vi "Read Servicio Seleccionado.vi"(8 "error in (no error)":errorcluster, 11 "Paquetes in":refnum<class "Paquetes.lvclass">) -> (0 "error out":errorcluster, 2 "Servicio Seleccionado":string, 3 "Paquetes out":refnum<class "Paquetes.lvclass">)   [LabVIEW 2020, in "Paquetes.lvlib" / "Paquetes.lvclass"]
uses:
  Paquetes.lvclass
  Paquetes.lvclass/Paquetes.ctl
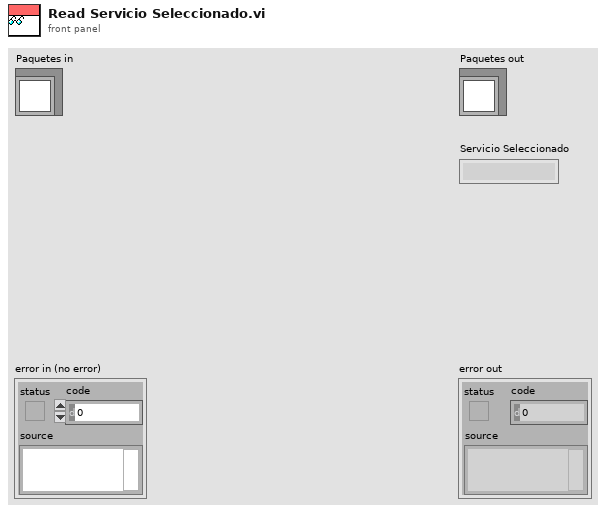
[diagram p1: front panel]
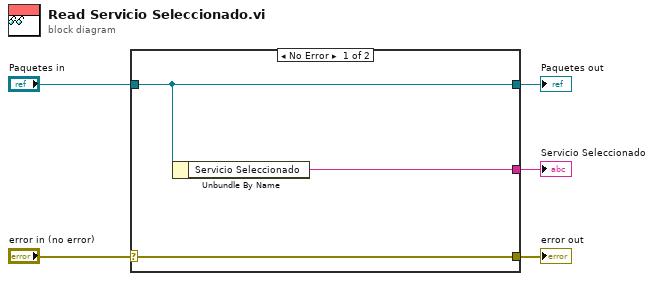
[diagram p0: block diagram]
diagram:
  n1 = case shown="No Error" "error in (no error)" {
    selector: "error in (no error)" -> [w8 w9]
    tunnel: [w8 w9] -> w4
    tunnel: [w7 w10] -> w2
    tunnel: "Paquetes in" -> [w7 w10]
    tunnel: [w6 _] -> w1
    frame No Error {
      n2 = Unbundle By Name(w7) -> ("Servicio Seleccionado"=w6:string)
    }
    frame Error {
    }
  }
  "error out" <- w4
  "Paquetes out" <- w2
  "Servicio Seleccionado" <- w1
